vi "Alarms.vi"(11 "Error":string) -> (1 "SensorLocked?":bool, 3 "Q_OutOfRange?":bool)   [LabVIEW 2020]
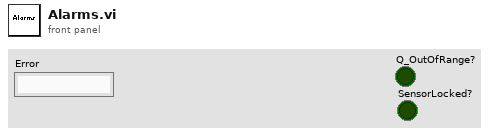
[diagram p1: front panel]
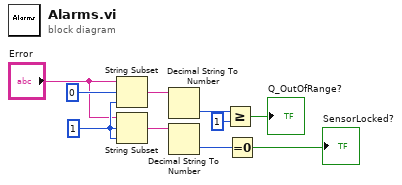
[diagram p0: block diagram]
diagram:
  w9 = 1 ("length (rest)")
  n1 = String Subset(string="Error", offset (0)=0, length (rest)=w9) -> (substring=w8:string)
  n2 = String Subset(string="Error", offset (0)=w9, length (rest)=w9) -> (substring=w7:string)
  n3 = Decimal String To Number(string=w8) -> (number=w6:i32)  [unwired: 2 in, 1 out]
  n4 = Decimal String To Number(string=w7) -> (number=w4:i32)  [unwired: 2 in, 1 out]
  n5 = Greater Or Equal?(x=w6, y=1) -> (x >= y?=→"Q_OutOfRange?":bool)
  n6 = Equal To 0?(x=w4) -> (x = 0?=→"SensorLocked?":bool)
